vi "add image.vi"(8 "error in (no error)":errorcluster caption="Fehler (Eingang, kein Fehler)", 9 "img.lvclass":refnum<class "img.lvclass">, 11 "Setup (Eingang)":refnum<class "Setup.lvclass">) -> (0 "error out":errorcluster caption="Fehler (Ausgang)", 3 "Setup (Ausgang)":refnum<class "Setup.lvclass">)   [LabVIEW 2013, in "DatenKlassen.lvlib" / "Setup.lvclass"]
uses:
  Setup.lvclass
  Image/img.lvclass
  Setup.lvclass/Setup.ctl
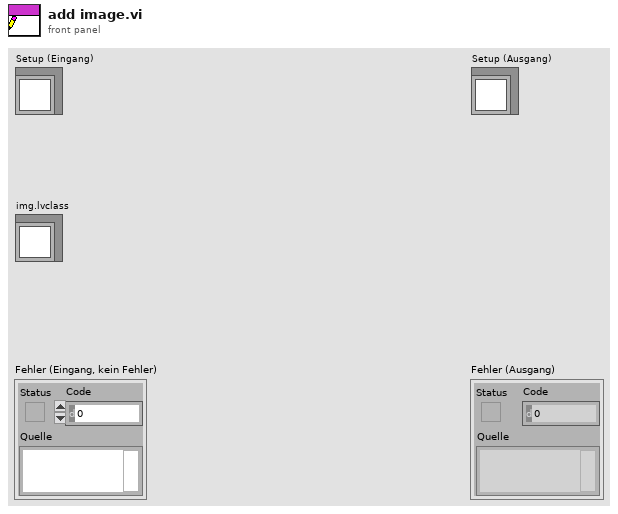
[diagram p1: front panel]
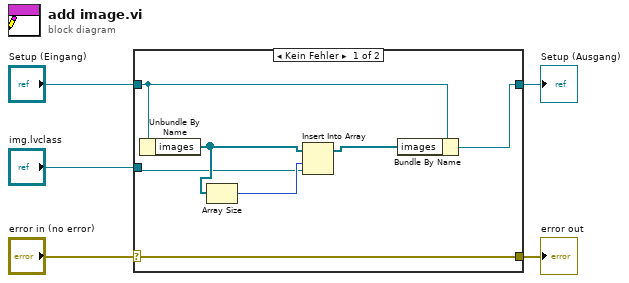
[diagram p0: block diagram]
diagram:
  n1 = case shown="Kein Fehler" "error in (no error)" {
    selector: "error in (no error)" -> [w12 w13]
    tunnel: [w12 w13] -> w4
    tunnel: [w11 w14] -> w2
    tunnel: "Setup (Eingang)" -> [w10 w14]
    tunnel: "img.lvclass" -> [w7 _]
    frame No Error {
      n2 = Unbundle By Name(w10) -> ("images"=w9:refnum<class "img.lvclass">[])
      n3 = Array Size(array=w9) -> (size(s)=w8:i32)
      n4 = Insert Into Array(array=w9, index=w8, new element=w7) -> (w6:refnum<class "img.lvclass">[])
      n5 = Bundle By Name(cluster=w10, "images"=w6) -> (w11:refnum<class "Setup.lvclass">)
    }
    frame Error {
    }
  }
  "error out" <- w4
  "Setup (Ausgang)" <- w2
